vi "SL2_AD_DLL_Phoibos_ListDataChannels.vi"(8 "error in":errorcluster, 9 "pHandle":u32, 11 "dll path in":path) -> (0 "error out":errorcluster, 1 "Channel_names":string[](array[string]), 2 "Channel_infos":T1[](array[typedef]), 3 "dll path out":path)   [LabVIEW 2020]
uses:
  DEFINITIONS/DEF_channel_info.ctl
  DEFINITIONS/DEF_T_error_enum.ctl
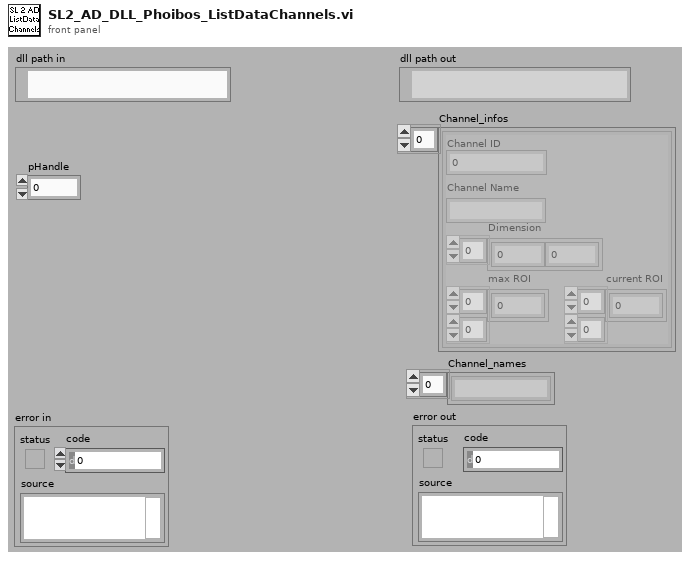
[diagram p1: front panel]
types:
  T1 = typedef "DEF_channel_info.ctl" = cluster{"Channel ID":u32, "Channel Name":string, "Dimension":u32[], "max ROI":u32[][], "current ROI":u32[][]}
  T2 = enum16{"open", "replace", "create", "open or create", "replace or create", "replace or create with confirmation"}
  T3 = typedef "DEF_T_error_enum.ctl" = u32
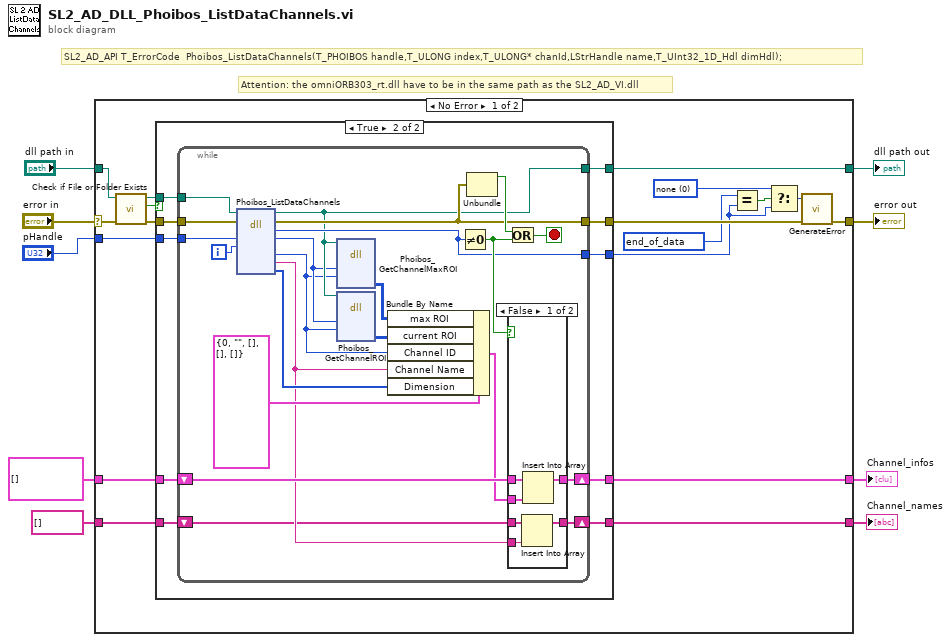
[diagram p0: block diagram]
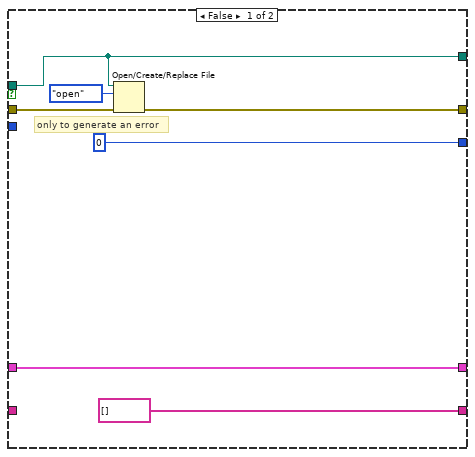
[diagram p2: hidden frame]
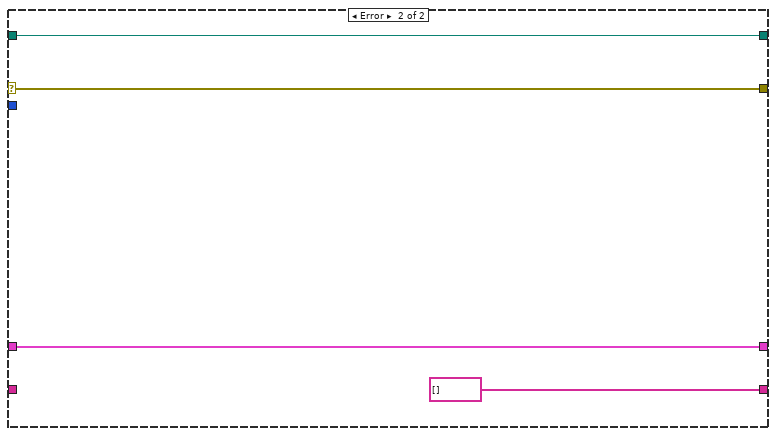
[diagram p4: hidden frame]
diagram:
  # "SL2_AD_API T_ErrorCode  Phoibos_ListDataChannels(T_PHOIBOS handle,T_ULONG index,T_ULONG* chanId,LStrHandle name,T_UInt32_1D_Hdl dimHdl);"
  # "Attention: the omniORB303_rt.dll have to be in the same path as the SL2_AD_VI.dll"
  n1 = case shown="No Error" "error in" {
    selector: "error in" -> [w26 w77]
    tunnel: [w18 w77] -> w9
    tunnel: [w27 w78] -> w8
    tunnel: "dll path in" -> [w25 w78]
    tunnel: "pHandle" -> [w24 _]
    tunnel: [w23 w76] -> w3
    tunnel: T1[] [] -> [w22 w76]
    tunnel: [w21 string[] []] -> w2
    tunnel: string[] [] -> [w20 _]
    frame No Error {
      w16 = T3 0 items=["none"=0, "busy"=65536, "error"=131072, "parameter"=262144, "locked"=524288, "sync"=1048576, "connection"=2097152, "internal"=4194304, "end_of_data"=8388608] ("DEF_T_error_enum")
      w15 = T3 8388608 items=["none"=0, "busy"=65536, "error"=131072, "parameter"=262144, "locked"=524288, "sync"=1048576, "connection"=2097152, "internal"=4194304, "end_of_data"=8388608] ("DEF_T_error_enum")
      n2 = call <vilib>:"Check if File or Folder Exists.vi"("error in (no error)"=w26, "path"=w25) -> ("error out"=w10:errorcluster, "file or folder exists?"=w12:bool, "dup path"=w11:path)  [unwired: 7 in]
      n3 = case shown="True" w12 {
        tunnel: [w32 w44] -> w19
        tunnel: [0 ("error_code") w43] -> w13
        tunnel: [w30 w42] -> w27
        tunnel: w11 -> [w30 w41]
        tunnel: w10 -> [w33 w40]
        tunnel: w24 -> [_ w39]
        tunnel: [w29 w38] -> w23
        tunnel: w22 -> [w29 w37]
        tunnel: [string[] [] w36] -> w21
        tunnel: w20 -> [_ w35]
        frame False {
          # "only to generate an error"
          n4 = Open/Create/Replace File(file path (use dialog)=w30, error in=w33, operation (0:open)=T2."open") -> (error out=w32:errorcluster)  [unwired: 3 in, 2 out]
        }
        frame True {
          n5 = while {
            tunnel: [w56] -> w43
            tunnel: [w60] -> w44
            tunnel: w41 -> [w59]
            tunnel: w40 -> [w61]
            tunnel: [w55] -> w42
            tunnel: w39 -> [w58]
            shift-right: [w62] -> w38
            shift-left: w37 -> [w63]
            shift-right: [w46] -> w36
            shift-left: w35 -> [w45]
            i -> [w57]
            stop <- w66 stop-if-true
            n6 = dll-call lib="C:/Programme/SPECS/SpecsLab2/programming/LabView7.1/SL2_AD_VI.dll" fn="Phoibos_ListDataChannels" ("GetChannelList")(path in=w59, error in=w61, "pHandle"=w58, "index"=w57) -> (path out=w55:path, error out=w60:errorcluster, "error_code"=w56:u32, "pHandle"=w54:u32, "chanId"=w49:u32, "name"=w47:string, "dim"=w48:u32[])  [unwired: 5 in]
            n7 = dll-call lib="C:/Programme/SPECS/SpecsLab2/programming/LabView7.1/SL2_AD_VI.dll" fn="Phoibos_GetChannelMaxROI" ("GetChannelMaxROI")(path in=w55, "handle"=w54, "chanId"=w49) -> ("roiArray2D"=w51:u32[][])  [unwired: 6 in, 2 out]
            n8 = dll-call lib="C:/Programme/SPECS/SpecsLab2/programming/LabView7.1/SL2_AD_VI.dll" fn="Phoibos_GetChannelROI" ("GetChannelROI")(path in=w55, "handle"=w54, "chanId"=w49) -> ("roiArray2D"=w50:u32[][])  [unwired: 6 in, 2 out]
            n9 = Bundle By Name(cluster=T1 {"Channel ID"=0, "Channel Name"="", "Dimension"=[], "max ROI"=[], "current ROI"=[]} ("DEF_Channel_info"), "max ROI"=w51, "current ROI"=w50, "Channel ID"=w49, "Channel Name"=w47, "Dimension"=w48) -> (w52:T1)
            n10 = Not Equal To 0?(x=w56) -> (x != 0?=w65:bool)
            n11 = Unbundle(w60) -> ("status"=w64:bool)  [unwired: 2 out]
            n12 = Or(x=w64, y=w65) -> (x .or. y?=w66:bool)
            n13 = case shown="False" w65 {
              tunnel: w52 -> [w72 _]
              tunnel: w63 -> [w71 w74]
              tunnel: [w70 w74] -> w62
              tunnel: w47 -> [w69 _]
              tunnel: [w68 w73] -> w46
              tunnel: w45 -> [w67 w73]
              frame False {
                n14 = Insert Into Array(array=w67, new element=w69) -> (w68:string[])  [unwired: 1 in]
                n15 = Insert Into Array(array=w71, new element=w72) -> (w70:T1[])  [unwired: 1 in]
              }
              frame True {
              }
            }
          }
        }
      }
      n16 = Equal?(x=w15, y=w13) -> (x = y?=w14:bool)
      n17 = Select(t=w16, s=w14, f=w13) -> (s? t:f=w17:T3)
      n18 = call "GenerateError.vi"("error in"=w19, "error_code"=w17) -> ("error out"=w18:errorcluster)  [unwired: 9 in]
    }
    frame Error {
    }
  }
  "error out" <- w9
  "dll path out" <- w8
  "Channel_infos" <- w3
  "Channel_names" <- w2
